vi "LoopPeriodGLOBAL (1).vi"() -> ()   [LabVIEW 2017]
panel:
  in  "Reed Switch Period (ms)":u32=2
  in  "IMU Period (ms)":u32=50
  in  "DAQ Period (ms)":u32=50
  in  "Control Period (10ms)":i64=1
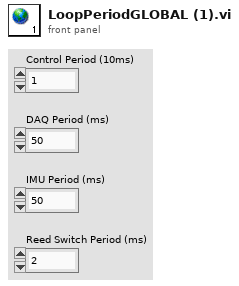
[diagram p1: front panel]
diagram:
